vi "Signal-status.vi"(6 "State":T1, 8 "error in (no error)":errorcluster, 11 "Data ref. in":refnum<data-value>) -> (0 "error out":errorcluster, 3 "Data ref.":refnum<data-value>)   [LabVIEW 2013, in "CameraVision.lvlib" / "CV-Main.lvclass"]
uses:
  CV-Main.lvclass
  Application-states.ctl
  CV-Main.lvclass/CV-Main.ctl
  Read Client.vi
  Write Status.vi
  Client/Sources/CV-Client.lvclass
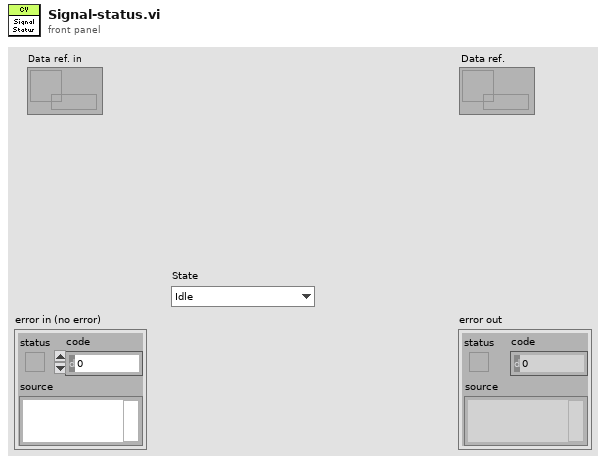
[diagram p1: front panel]
types:
  T1 = typedef "CameraVision.lvlib/CV-Main.lvclass/Application-states.ctl" = enum16{"Idle", "Initialized", "Configured", "Activated", "Started", "Stopped", "Reset", "Error", "Exited"}
  T2 = typedef "CameraVision.lvlib/CV-Client.lvclass/Object-reference.ctl" = refnum<data-value>
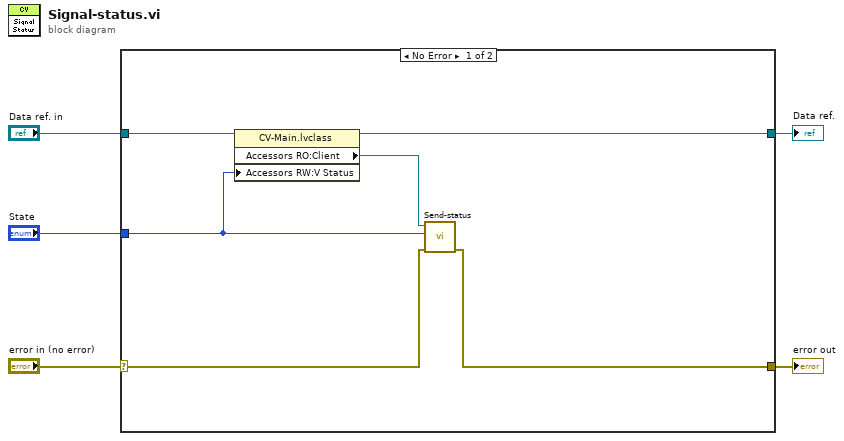
[diagram p0: block diagram]
diagram:
  n1 = case shown="No Error" "error in (no error)" {
    selector: "error in (no error)" -> [w9 w13]
    tunnel: [w8 w13] -> w4
    tunnel: "Data ref. in" -> [w11 w12]
    tunnel: [w7 w12] -> w2
    tunnel: "State" -> [w6 _]
    frame No Error {
      n2 = property class="CV-Main.lvclass"(reference=w11, "Accessors RW:V Status"=w6) -> (reference out=w7:refnum<data-value>, "Accessors RO:Client"=w10:T2)  [unwired: 1 in, 1 out]
      n3 = call "Send-status.vi"("error in (no error)"=w9, "Status"=w6, "Client in"=w10) -> ("error out"=w8:errorcluster)  [unwired: 7 in, 1 out]
    }
    frame Error {
    }
  }
  "error out" <- w4
  "Data ref." <- w2
